vi "GET_Gaussian_kernel.vi"(8 "Error In":errorcluster, 9 "Sigma":dbl=1.0, 10 "Interp. steps":i32=25, 11 "Kernel size":u32=5) -> (0 "Error Out":errorcluster, 3 "Gaussian kernel (normalized)":dbl[][](array[numeric]))   [LabVIEW 2018, in "Tracker.lvlib"]
uses:
  Tracker.lvlib
panel:
  out "Coord template":dbl[](array[numeric])
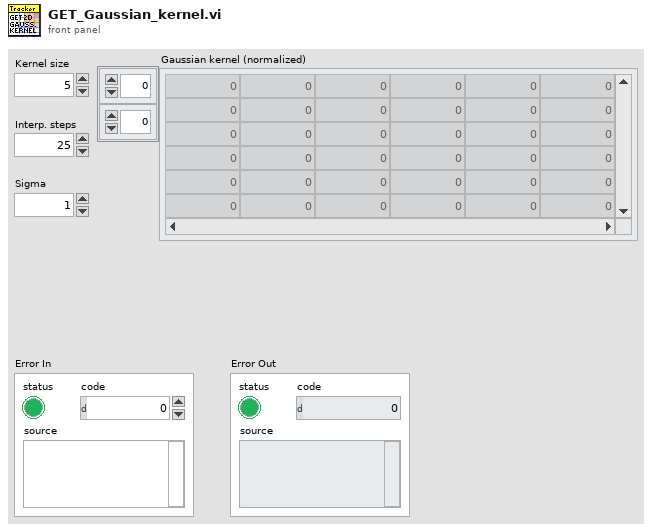
[diagram p1: front panel]
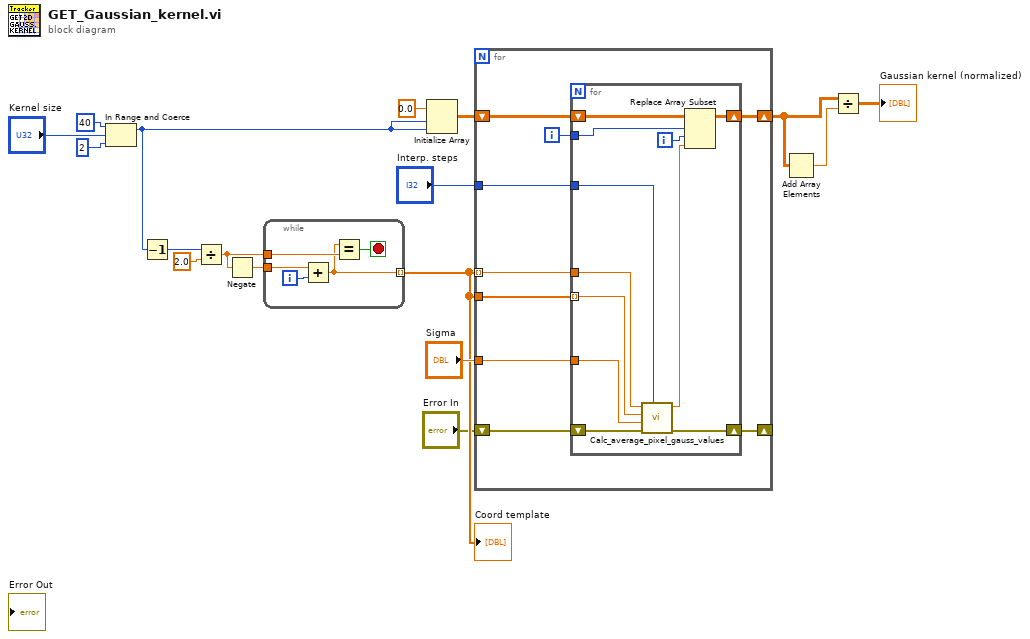
[diagram p0: block diagram]
diagram:
  n1 = In Range and Coerce(upper limit=u32 40, x="Kernel size", lower limit=u32 2) -> (coerced(x)=w7:u32)  [unwired: 1 out]
  n2 = Decrement(x=w7) -> (x-1=w11:u32)
  n3 = Divide(x=w11, y=2.0) -> (x/y=w12:dbl)
  n4 = Negate(x=w12) -> (-x=w14:dbl)
  n5 = while {
    tunnel: w14 -> [w22]
    tunnel: w12 -> [w20]
    tunnel: [w18] -> w6 mode=indexing
    i -> [w21]
    stop <- w19 stop-if-true
    n6 = Add(x=w22, y=w21) -> (x+y=w18:dbl)
    n7 = Equal?(x=w18, y=w20) -> (x = y?=w19:bool)
  }
  "Coord template" <- w6
  n8 = Initialize Array(0.0 ("element"), w7, w7) -> (w9:dbl[][])
  n9 = for {
    tunnel: w6 -> [w30] mode=indexing
    tunnel: "Sigma" -> [w29]
    shift-right: [w27] -> w3
    shift-left: w9 -> [w31]
    tunnel: w6 -> [w26]
    tunnel: "Interp. steps" -> [w25]
    shift-right: [w23] -> _
    shift-left: "Error In" -> [w24]
    i -> [w28]
    n10 = for {
      tunnel: w30 -> [w42]
      tunnel: w29 -> [w41]
      tunnel: w28 -> [w39]
      shift-right: [w36] -> w27
      shift-left: w31 -> [w40]
      tunnel: w26 -> [w35] mode=indexing
      tunnel: w25 -> [w32]
      shift-right: [w33] -> w23
      shift-left: w24 -> [w34]
      i -> [w38]
      n11 = call "Calc_average_pixel_gauss_values.vi"("Interp. steps"=w32, "error in (no error)"=w34, "Sigma"=w41, "Y"=w35, "X"=w42) -> ("error out"=w33:errorcluster, "Average interp. gaussian value"=w37:dbl)  [unwired: 4 in, 1 out]
      n12 = Replace Array Subset(array=w40, new element=w37, index (row)=w39, index (col)=w38) -> (w36:dbl[][])
    }
  }
  n13 = Add Array Elements(numeric array=w3) -> (sum=w2:dbl)
  n14 = Divide(x=w3, y=w2) -> (x/y=→"Gaussian kernel (normalized)":dbl[][])
